vi "StatisticalData2.vi"() -> ()   [LabVIEW 2018]
uses:
  <vilib>/Utility/config.llb/Read Key (Double).vi
  <vilib>/Utility/config.llb/NI_LVConfig.lvlib
panel:
  in  "configuration file path":path caption="配置文件的路径"
  out "字符串数组":string[](array[string])
  out "双精度数组":dbl[](array[numeric])
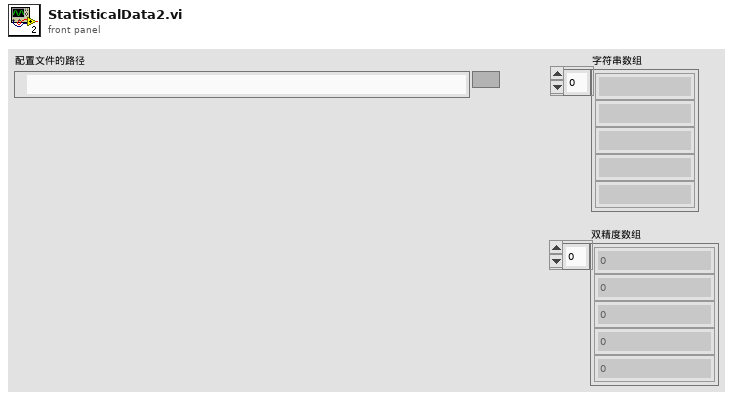
[diagram p1: front panel]
types:
  T1 = typedef "NI_LVConfig.lvlib/Config Data RefNum.ctl" = refnum<k1>
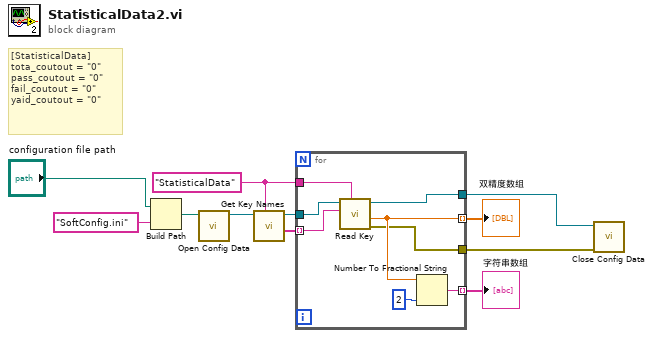
[diagram p0: block diagram]
diagram:
  w3 = "StatisticalData" ("section")
  # "[StatisticalData]\ntota_coutout = \"0\"\npass_coutout = \"0\"\nfail_coutout = \"0\"\nyaid_coutout = \"0\""
  n1 = Build Path(base path="configuration file path", name or relative path="SoftConfig.ini" ("名称或相对路径")) -> (appended path=w9:path)
  n2 = call <vilib>:"Open Config Data.vi"("configuration file path"=w9) -> ("refnum"=w1:T1)  [unwired: 8 in, 2 out]
  n3 = call <vilib>:"Get Key Names.vi"("section"=w3, "refnum"=w1) -> ("key names"=w2:string[], "refnum out"=w4:T1)  [unwired: 6 in, 2 out]
  n4 = for {
    tunnel: w2 -> [w18] mode=indexing
    tunnel: w3 -> [w19]
    tunnel: w4 -> [w17]
    tunnel: [w16] -> w5 mode=indexing
    tunnel: [w14] -> w6 mode=indexing
    tunnel: [w13] -> w10
    tunnel: [w12] -> w11
    n5 = call-poly <vilib>:"Read Key.vi"("section"=w19, "key"=w18, "refnum"=w17) -> ("error out"=w12:errorcluster, "value"=w16:dbl, "refnum out"=w13:T1)  [unwired: 5 in, 1 out]
    n6 = Number To Fractional String(number=w16, precision (6)=i16 2 ("精度(6)")) -> (F-format string=w14:string)  [unwired: 2 in]
  }
  "字符串数组" <- w6
  "双精度数组" <- w5
  n7 = call <vilib>:"Close Config Data.vi"("error in (no error)"=w11, "refnum"=w10) -> ()  [unwired: 8 in, 2 out]
